vi "TwrBotInputScale.vi"(0 "Signal (V)":dbl, 9 "Scale (Nm/V)":dbl, 11 "Offset (Nm)":dbl) -> (4 "Output (Nm)":dbl)   [LabVIEW 2018]
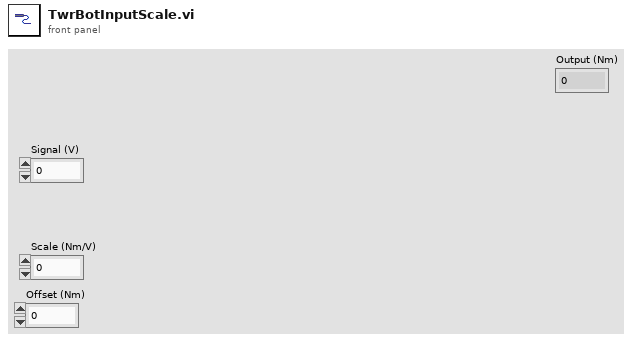
[diagram p1: front panel]
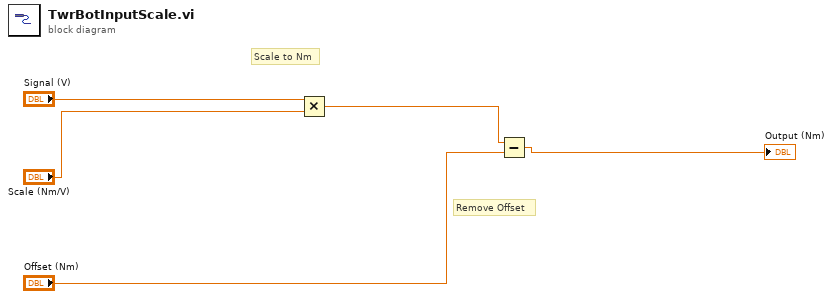
[diagram p0: block diagram]
diagram:
  # "Scale to Nm"
  # "Remove Offset"
  n1 = Multiply(x="Signal (V)", y="Scale (Nm/V)") -> (x*y=w3:dbl)
  n2 = Subtract(x=w3, y="Offset (Nm)") -> (x-y=→"Output (Nm)":dbl)
